vi "Queue Driver_Sender.vi"(0 "Array of States":cluster{"State":string, "Data":variant}[](array[cluster]), 2 "Queue Name":string, 11 "Error In":errorcluster, 13 "Operation":T1) -> (4 "Data Cluster":cluster{"State":string, "Data":variant}, 15 "Error Out":errorcluster)   [LabVIEW 2020, in "Data Communication Transmitter.lvlib"]
doc: "Queue Driver to store the sender's states."
uses:
  Data Communication Transmitter.lvlib
  Typedefs/Queue Operation_Sender.ctl
panel:
  # "Queue driver"
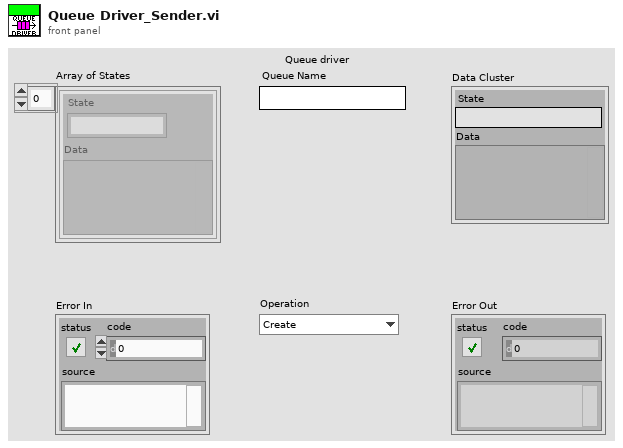
[diagram p1: front panel]
types:
  T1 = typedef "Data Communication Transmitter.lvlib/Queue Operation_Sender.ctl" = enum16{"Create", "Enqueue", "Enstack", "Dequeue", "Flush", "Release"}
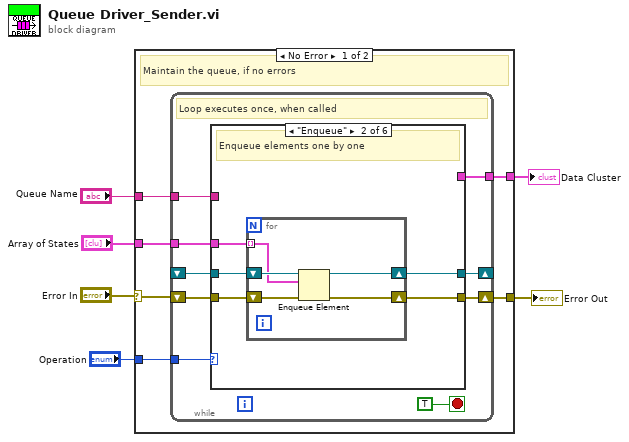
[diagram p0: block diagram]
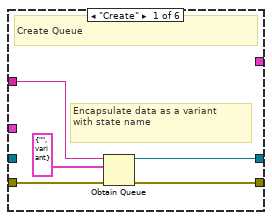
[diagram p2: hidden frame]
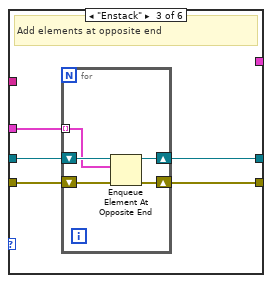
[diagram p3: hidden frame]
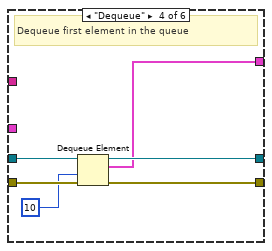
[diagram p4: hidden frame]
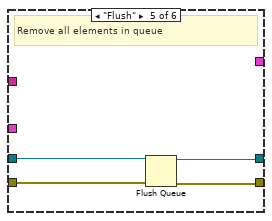
[diagram p5: hidden frame]
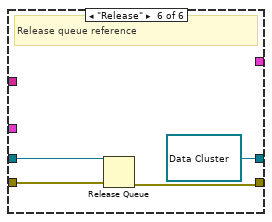
[diagram p6: hidden frame]
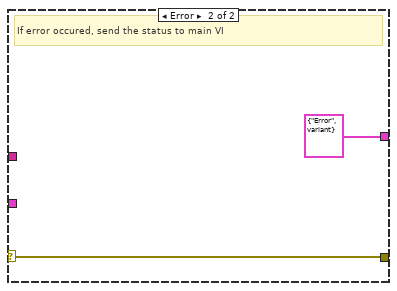
[diagram p7: hidden frame]
diagram:
  n1 = case shown="No Error" "Error In" {
    selector: "Error In" -> [w12 w62]
    tunnel: [w11 w62] -> w5
    tunnel: "Operation" -> [w10 _]
    tunnel: "Queue Name" -> [w9 _]
    tunnel: "Array of States" -> [w8 _]
    tunnel: [w7 cluster{"State":string, "Data":variant} {"State"="Error", "Data"=variant} ("Data Cluster")] -> w1
    frame No Error {
      # "Maintain the queue, if no errors"
      n2 = while {
        shift-right: [w19] -> w11
        shift-left: w12 -> [w20]
        tunnel: w10 -> [w18]
        tunnel: w9 -> [w17]
        tunnel: w8 -> [w16]
        shift-right: [w15] -> _
        shift-left: _ -> [w14]
        tunnel: [w13] -> w7
        stop <- TRUE stop-if-true
        # "Loop executes once, when called"
        n3 = case shown="\"Enqueue\"" w18 {
          tunnel: w20 -> [w26 w28 w40 w52 w56 w60]
          tunnel: [w25 w29 w39 w51 w53 w59] -> w19
          tunnel: w17 -> [w24 _ _ _ _ _]
          tunnel: w16 -> [_ w27 w37 _ _ _]
          tunnel: [w23 w30 w38 w49 w54 refnum<queue> refnum ("queue out")] -> w15
          tunnel: w14 -> [_ w31 w41 w50 w55 w57]
          tunnel: [_ _ _ w48 _ _] -> w13
          frame "Create" {
            # "Encapsulate data as a variant\nwith state name"
            # "Create Queue"
            n4 = Obtain Queue(name (unnamed)=w24, element data type=cluster{"State":string, "Data":variant} {"State"="", "Data"=variant} ("Data Cluster"), error in (no error)=w26) -> (queue out=w23:refnum<queue>, error out=w25:errorcluster)  [unwired: 2 in, 1 out]
          }
          frame "Enqueue" {
            # "Enqueue elements one by one"
            n5 = for {
              shift-right: [w34] -> w29
              shift-left: w28 -> [w33]
              tunnel: w27 -> [w32] mode=indexing
              shift-right: [w35] -> w30
              shift-left: w31 -> [w36]
              n6 = Enqueue Element(queue=w36, element=w32, error in (no error)=w33) -> (queue out=w35:refnum<queue>, error out=w34:errorcluster)  [unwired: 1 in, 1 out]
            }
          }
          frame "Enstack" {
            # "Add elements at opposite end"
            n7 = for {
              shift-right: [w45] -> w39
              shift-left: w40 -> [w44]
              tunnel: w37 -> [w42] mode=indexing
              shift-right: [w46] -> w38
              shift-left: w41 -> [w43]
              n8 = Enqueue Element At Opposite End(queue=w43, element=w42, error in (no error)=w44) -> (queue out=w46:refnum<queue>, error out=w45:errorcluster)  [unwired: 1 in, 1 out]
            }
          }
          frame "Dequeue" {
            # "Dequeue first element in the queue"
            n9 = Dequeue Element(queue=w50, timeout in ms (-1)=10, error in (no error)=w52) -> (queue out=w49:refnum<queue>, element=w48:cluster{"State":string, "Data":variant}, error out=w51:errorcluster)  [unwired: 1 out]
          }
          frame "Flush" {
            # "Remove all elements in queue"
            n10 = Flush Queue(queue=w55, error in (no error)=w56) -> (queue out=w54:refnum<queue>, error out=w53:errorcluster)  [unwired: 1 out]
          }
          frame "Release" {
            # "Release queue reference"
            n11 = Release Queue(queue=w57, error in (no error)=w60) -> (error out=w59:errorcluster)  [unwired: 1 in, 2 out]
          }
        }
      }
    }
    frame Error {
      # "If error occured, send the status to main VI"
    }
  }
  "Error Out" <- w5
  "Data Cluster" <- w1
